vi "Ex7.vi"() -> ()   [LabVIEW 2016]
uses:
  <vilib>/DAQmx/write.llb/DAQmx Write (Analog 1D Wfm NChan NSamp).vi
  <vilib>/DAQmx/read.llb/DAQmx Read (Analog 1D Wfm NChan NSamp).vi
  <vilib>/DAQmx/create/channels.llb/DAQmx Create Channel (AI-Voltage-Basic).vi
  <vilib>/DAQmx/configure/trigger.llb/DAQmx Start Trigger (Digital Edge).vi
  <vilib>/DAQmx/create/channels.llb/DAQmx Create Channel (AO-Voltage-Basic).vi
  <vilib>/DAQmx/configure/timing.llb/DAQmx Timing (Sample Clock).vi
  <vilib>/DAQmx/miscellaneous.llb/DAQmx Fill In Error Info.vi
  <vilib>/measure/NI_MABase.lvlib
panel:
  in  "number of samples per channel":i32=1000
  out "웨이브폼 그래프 2":waveform(dbl)[](graph)
  in  "정지":bool
  out "웨이브폼 그래프":waveform(dbl)[](graph)
  in  "숫자형":dbl
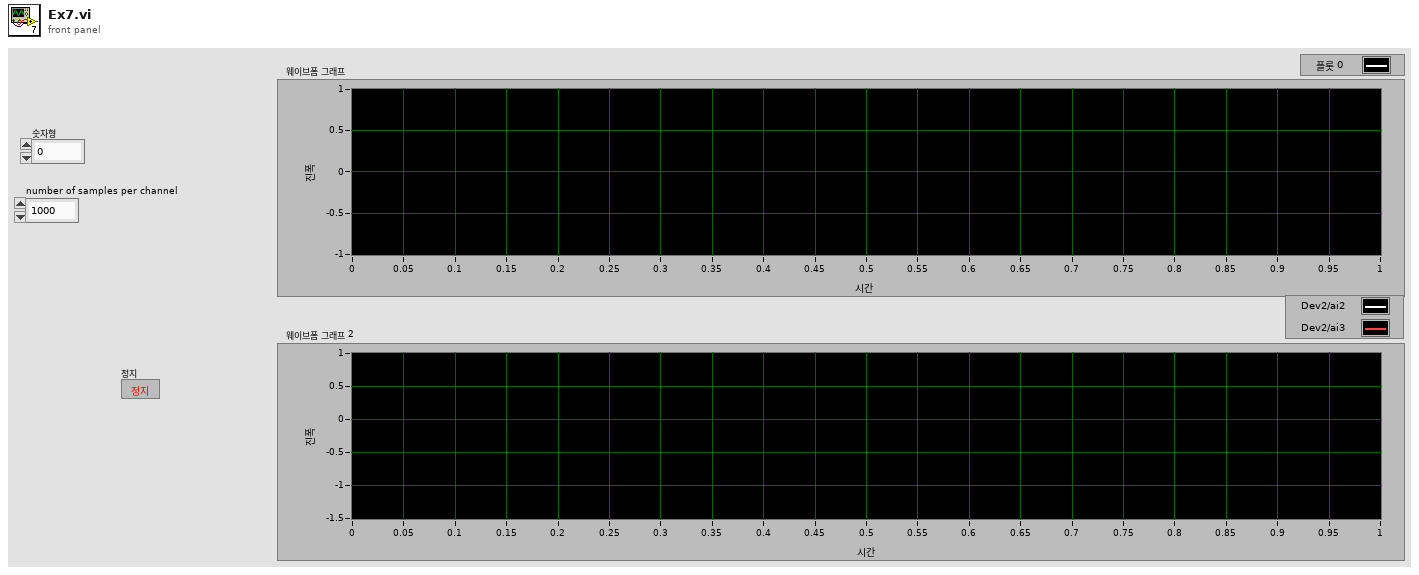
[diagram p1: front panel]
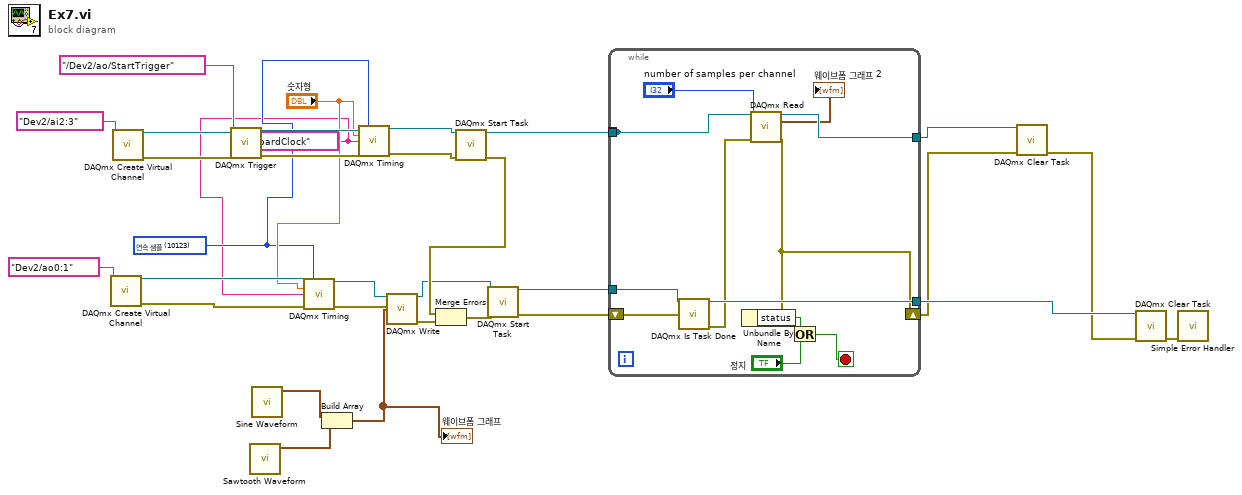
[diagram p0: block diagram]
diagram:
  w1 = tag "OnboardClock" ("source")
  w2 = 10123 items=["유한 샘플"=10178, "연속 샘플"=10123, "하드웨어 타이밍에 의한 단일 포인트"=12522] ("sample mode")
  n1 = call-poly <vilib>:"DAQmx Create Virtual Channel.vi"("physical channels"=tag "Dev2/ao0:1") -> ("task out"=w23:refnum<k21>, "error out"=w22:errorcluster)  [unwired: 13 in]
  n2 = call-poly <vilib>:"DAQmx Create Virtual Channel.vi"("physical channels"=tag "Dev2/ai2:3") -> ("task out"=w21:refnum<k21>, "error out"=w30:errorcluster)  [unwired: 13 in]
  n3 = call-poly <vilib>:"DAQmx Trigger.vi"("task/channels in"=w21, "source"=tag "/Dev2/ao/StartTrigger", "error in"=w30) -> ("task out"=w28:refnum<k21>, "error out"=w27:errorcluster)  [unwired: 11 in]
  n4 = call <vilib>:"Sawtooth Waveform.vi"() -> ("signal out"=w9:waveform(dbl))  [unwired: 10 in, 1 out]
  n5 = call <vilib>:"Sine Waveform.vi"() -> ("signal out"=w10:waveform(dbl))  [unwired: 10 in, 1 out]
  n6 = call-poly <vilib>:"DAQmx Timing.vi"("task/channels in"=w23, "sample mode"=w2, "rate"="숫자형", "source"=w1, "error in"=w22) -> ("task out"=w12:refnum<k21>, "error out"=w19:errorcluster)  [unwired: 9 in]
  n7 = Build Array(w10, w9) -> (w8:waveform(dbl)[])
  "웨이브폼 그래프" <- w8
  n8 = call-poly <vilib>:"DAQmx Timing.vi"("task/channels in"=w28, "sample mode"=w2, "rate"="숫자형", "source"=w1, "error in"=w27) -> ("task out"=w26:refnum<k21>, "error out"=w25:errorcluster)  [unwired: 9 in]
  n9 = call-poly <vilib>:"DAQmx Write.vi"("task/channels in"=w12, "data"=w8, "error in"=w19) -> ("task out"=w11:refnum<k21>, "error out"=w13:errorcluster)  [unwired: 10 in, 1 out]
  n10 = call <vilib>:"DAQmx Start Task.vi"("task/channels in"=w26, "error in"=w25) -> ("task out"=w15:refnum<k21>, "error out"=w17:errorcluster)  [unwired: 12 in]
  n11 = Merge Errors(w17, w13) -> (w18:errorcluster)
  n12 = call <vilib>:"DAQmx Start Task.vi"("task/channels in"=w11, "error in"=w18) -> ("task out"=w14:refnum<k21>, "error out"=w16:errorcluster)  [unwired: 12 in]
  n13 = while {
    tunnel: [w40] -> _
    tunnel: w15 -> [w40]
    tunnel: w14 -> [w43]
    shift-right: [w35] -> w6
    shift-left: w16 -> [w42]
    tunnel: [w41] -> w7
    tunnel: [w39] -> w3
    stop <- w36 stop-if-true
    n14 = call <vilib>:"DAQmx Is Task Done.vi"("task/channels in"=w43, "error in"=w42) -> ("task out"=w41:refnum<k21>, "error out"=w34:errorcluster)  [unwired: 11 in, 1 out]
    n15 = call-poly <vilib>:"DAQmx Read.vi"("task/channels in"=w40, "number of samples per channel"="number of samples per channel", "error in"=w34) -> ("task out"=w39:refnum<k21>, "data"=→"웨이브폼 그래프 2":waveform(dbl)[], "error out"=w35:errorcluster)  [unwired: 10 in]
    n16 = Unbundle By Name(w35) -> ("status"=w38:bool)
    n17 = Or(x=w38, y="정지") -> (x .or. y?=w36:bool)
  }
  n18 = call <vilib>:"DAQmx Clear Task.vi"("task in"=w3, "error in"=w6) -> ("error out"=w5:errorcluster)  [unwired: 13 in]
  n19 = call <vilib>:"DAQmx Clear Task.vi"("task in"=w7, "error in"=w5) -> ("error out"=w4:errorcluster)  [unwired: 13 in]
  n20 = call <vilib>:"Simple Error Handler.vi"("error in (no error)"=w4) -> ()  [unwired: 4 in, 5 out]
